vi "启动流程.vi"   [LabVIEW 2016, in "综合生物毒性.lvlib"]
types:
  T1 = cluster{"连接类型":enum16{"串口", "TCP"}, "串口":string, "IP":string, "PORT":string}
  T2 = cluster{"时间标识":timestamp, "设备":string, "日志信息":string, "流程参数":string}
  T3 = cluster{"时间标识":timestamp, "测量模式":string, "数据类型":string, "监测值":sgl, "单位":string, "数据标识":string, "因子编码":string, "标样参考值":sgl}
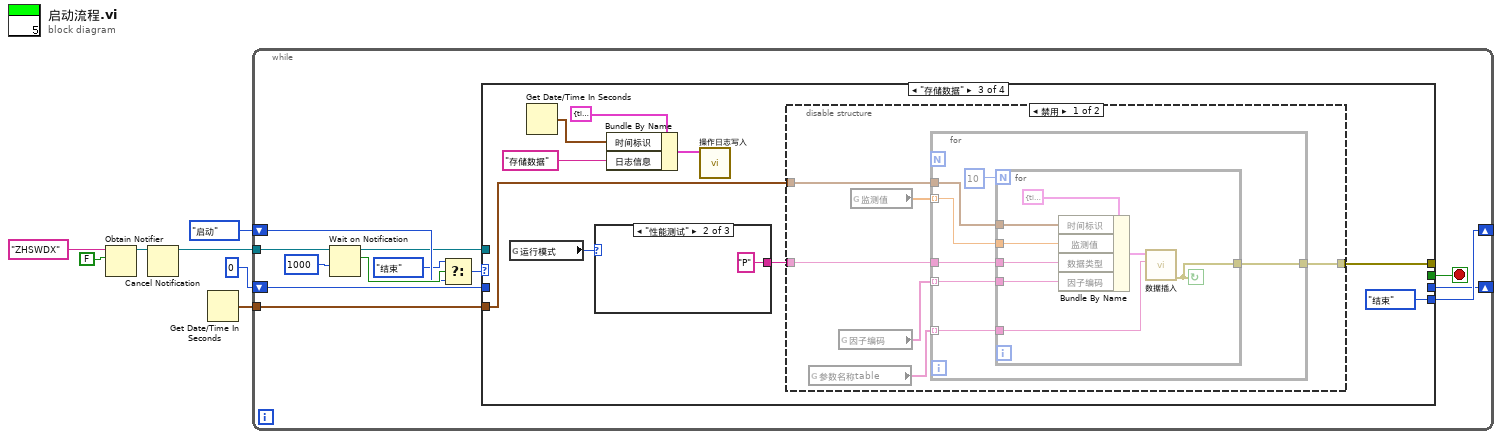
[diagram p0: block diagram]
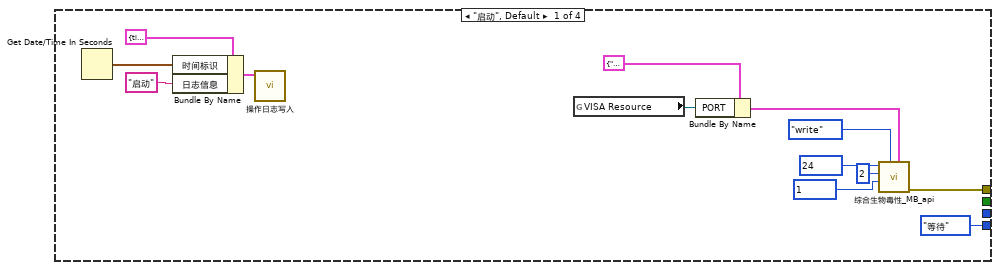
[diagram p2: hidden frame]
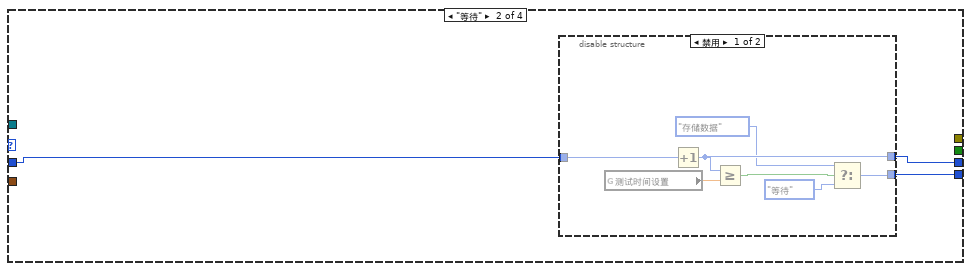
[diagram p3: hidden frame]
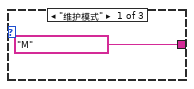
[diagram p6: hidden frame]
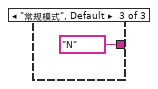
[diagram p7: hidden frame]
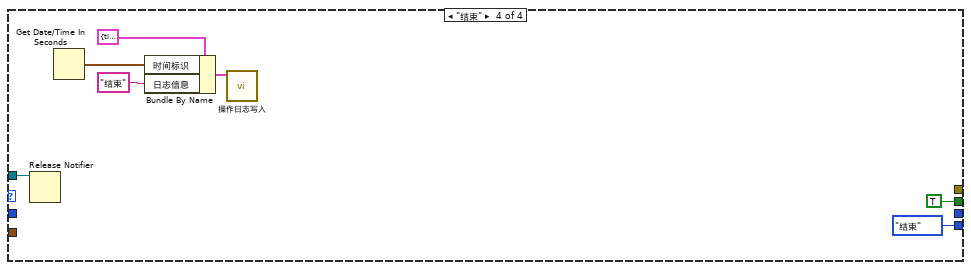
[diagram p8: hidden frame]
diagram:
  n1 = Obtain Notifier(name (unnamed)="ZHSWDX" ("名称（未命名）"), notification data type=FALSE) -> (notifier out=w2:refnum<notifier>)  [unwired: 2 in, 2 out]
  n2 = Cancel Notification(0:w2) -> (8:w1:refnum<notifier>)  [unwired: 1 in, 2 out]
  n3 = Get Date/Time In Seconds() -> (seconds since 1Jan1904=w5:timestamp)
  n4 = while {
    shift-right: [w19] -> _
    shift-left: enum16{"启动", "等待", "存储数据", "结束"}."启动" ("枚举") -> [w11]
    shift-right: [w17] -> _
    shift-left: u32 0 ("等待时间（毫秒）") -> [w18]
    tunnel: w5 -> [w15]
    tunnel: w1 -> [w14]
    stop <- w16 stop-if-true
    n5 = Wait on Notification(notifier=w14, timeout in ms (-1)=1000 ("超时毫秒(-1)")) -> (notifier out=w8:refnum<notifier>, notification=w12:bool)  [unwired: 2 in, 2 out]
    n6 = Select(t=enum16{"启动", "等待", "存储数据", "结束"}."结束", s=w12, f=w11) -> (s? t:f=w10:enum16{"启动", "等待", "存储数据", "结束"})
    n7 = case shown="\"存储数据\"" w10 {
      tunnel: [w32 _ w44 _] -> _
      tunnel: [enum16{"启动", "等待", "存储数据", "结束"}."等待" ("枚举") w33 enum16{"启动", "等待", "存储数据", "结束"}."结束" ("枚举") enum16{"启动", "等待", "存储数据", "结束"}."结束" ("枚举")] -> w19
      tunnel: w18 -> [_ w35 _ _]
      tunnel: [_ w34 _ _] -> w17
      tunnel: [_ _ _ TRUE] -> w16
      tunnel: w15 -> [_ _ w43 _]
      tunnel: w8 -> [_ _ _ w76]
      frame "启动", Default {
        n8 = Get Date/Time In Seconds() -> (seconds since 1Jan1904=w28:timestamp)
        n9 = Bundle By Name(cluster=T2 {"时间标识"=timestamp(0 s since 1904-01-01), "设备"="重金属", "日志信息"="", "流程参数"=""} ("data in"), "时间标识"=w28, "日志信息"="启动") -> (w29:T2)
        n10 = call "操作日志写入.vi"("data in"=w29) -> ()  [unwired: 10 in, 1 out]
        n11 = global read "全局_综合生物毒性.vi" "VISA Resource"() -> (w21:refnum<visa-resource-name>)
        n12 = Bundle By Name(cluster=T1 {"连接类型"=enum."串口", "串口"="", "IP"="192.168.1.205", "PORT"="502"} ("连接配置"), "PORT"=w21) -> (w20:T1)
        n13 = call "综合生物毒性_MB_api.vi"("连接配置"=w20, "STEP"=enum16{"open", "read", "write", "close"}."write", "values"=u16 1 ("starting address"), "quantity"=u16 2, "starting address"=u16 24) -> ("error out"=w32:errorcluster)  [unwired: 3 in, 3 out]
      }
      frame "等待" {
        n14 = disable-structure shown="禁用" {
          disable-tunnel: w35 -> [w42 _]
          disable-tunnel: [w41 _] -> w34
          disable-tunnel: [w38 _] -> w33
          frame Disabled {
            n15 = global read "全局变量.vi" "测试时间设置"() -> (w36:dbl)
            n16 = Increment(x=w42) -> (x+1=w41:u32)
            n17 = Greater Or Equal?(x=w41, y=w36) -> (x >= y?=w40:bool)
            n18 = Select(t=enum16{"启动", "等待", "存储数据", "结束"}."存储数据" ("枚举"), s=w40, f=enum16{"启动", "等待", "存储数据", "结束"}."等待" ("枚举")) -> (s? t:f=w38:enum16{"启动", "等待", "存储数据", "结束"})
          }
          frame Enabled {
          }
        }
      }
      frame "存储数据" {
        n19 = global read "全局变量.vi" "运行模式"() -> (w45:enum16{"维护模式", "常规模式", "应急模式", "质控模式", "性能测试"})
        n20 = Get Date/Time In Seconds() -> (seconds since 1Jan1904=w48:timestamp)
        n21 = case shown="\"性能测试\"" w45 {
          tunnel: ["M" ("数据标记表") "P" ("数据标记表") "N" ("数据标记表")] -> w46
          frame "维护模式" {
          }
          frame "性能测试" {
          }
          frame "常规模式", Default {
          }
        }
        n22 = Bundle By Name(cluster=T2 {"时间标识"=timestamp(0 s since 1904-01-01), "设备"="重金属", "日志信息"="", "流程参数"=""} ("data in"), "时间标识"=w48, "日志信息"="存储数据") -> (w49:T2)
        n23 = call "操作日志写入.vi"("data in"=w49) -> ()  [unwired: 10 in, 1 out]
        n24 = disable-structure shown="禁用" {
          disable-tunnel: w46 -> [w57 _]
          disable-tunnel: [w56 _] -> w44
          disable-tunnel: w43 -> [w55 _]
          frame Disabled {
            n25 = global read "全局变量.vi" "参数名称table"() -> (w54:string[])
            n26 = global read "全局变量.vi" "因子编码"() -> (w53:string[])
            n27 = global read "全局变量.vi" "监测值"() -> (w52:dbl[])
            n28 = for {
              tunnel: w52 -> [w63] mode=indexing
              tunnel: w57 -> [w64]
              tunnel: [w62] -> w56
              tunnel: w55 -> [w61]
              tunnel: w53 -> [w60] mode=indexing
              tunnel: w54 -> [w59] mode=indexing
              n29 = for {
                N: 10 -> [_]
                tunnel: w64 -> [w72]
                tunnel: w63 -> [w71]
                tunnel: [w65] -> w62
                tunnel: w61 -> [w70]
                tunnel: w60 -> [w69]
                tunnel: w59 -> [w68]
                stop <- w65 continue-if-true
                n30 = Bundle By Name(cluster=T3 {"时间标识"=timestamp(0 s since 1904-01-01), "测量模式"="水样测试", "数据类型"="N", "监测值"=0.0, "单位"="mg/L", "数据标识"="N", "因子编码"="w20122", "标样参考值"=0.0} ("data"), "时间标识"=w70, "监测值"=w71, "数据类型"=w72, "因子编码"=w69) -> (w67:T3)
                n31 = call "数据插入.vi"("table"=w68, "data"=w67) -> ("error out"=w65:errorcluster)  [unwired: 9 in]
              }
            }
          }
          frame Enabled {
          }
        }
      }
      frame "结束" {
        n32 = Release Notifier(notifier=w76) -> ()  [unwired: 2 in, 3 out]
        n33 = Get Date/Time In Seconds() -> (seconds since 1Jan1904=w78:timestamp)
        n34 = Bundle By Name(cluster=T2 {"时间标识"=timestamp(0 s since 1904-01-01), "设备"="重金属", "日志信息"="", "流程参数"=""} ("data in"), "时间标识"=w78, "日志信息"="结束") -> (w79:T2)
        n35 = call "操作日志写入.vi"("data in"=w79) -> ()  [unwired: 10 in, 1 out]
      }
    }
  }
